vi "globalSetUp.vi"(8 "error in":errorcluster, 11 "Deployment in":refnum<class "Deployment.lvclass">) -> (0 "error out":errorcluster, 3 "Deployment out":refnum<class "Deployment.lvclass">)   [LabVIEW 2020, in "Deployment.lvclass"]
uses:
  Deployment.lvclass
  Shared/Device Parameters.ctl
  Shared/Initialization Method.ctl
  Shared/Bus Selection.ctl
  Shared/Coupling Mode.ctl
  Deployment.lvclass/Deployment.ctl
  niveristand-custom-device-testing-tools/VeriStandTestUtilities/VeriStandTestUtilities.lvlib
  Scripting/AIM MIL-STD-1553 Scripting.lvlib
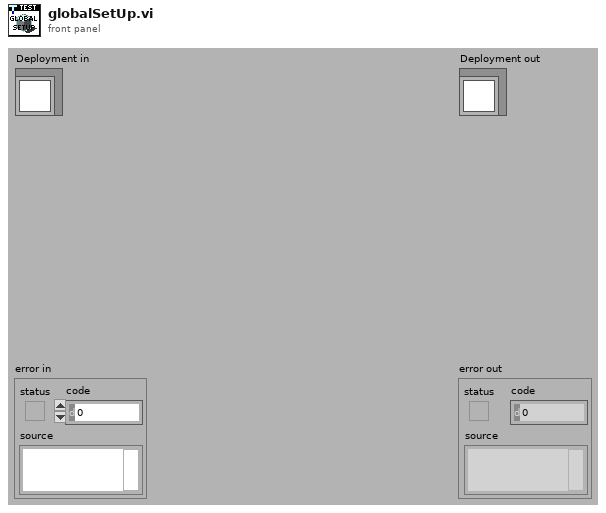
[diagram p1: front panel]
types:
  T1 = typedef "Device Parameters.ctl" = cluster{"initialization method":T2, "card number":i32, "pxi slot number":i32, "biu number":i32, "bus selection":T3, "coupling mode":T4}
  T2 = typedef "Initialization Method.ctl" = enum16{"PXI Slot Number", "Card Number"}
  T3 = typedef "Bus Selection.ctl" = enum16{"Both", "Primary", "Secondary"}
  T4 = typedef "Coupling Mode.ctl" = enum16{"Isolated Onboard Termination", "Transformer Coupled", "Direct Coupled", "External with Onboard Termination", "Onboard Digital Wrap-around"}
  T5 = typedef "Custom Device API.lvlib/Custom Device Item Ref.ctl" = u64
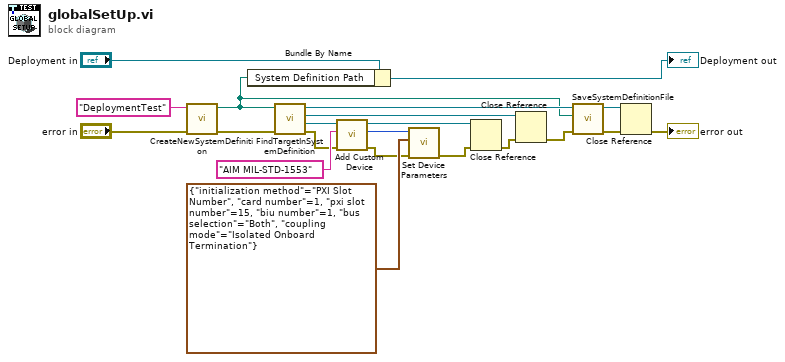
[diagram p0: block diagram]
diagram:
  n1 = call "CreateNewSystemDefinition.vi"("error in"="error in", "System Definition Name"="DeploymentTest") -> ("error out"=w5:errorcluster, "System Definition Path"=w7:path)  [unwired: 8 in]
  n2 = Bundle By Name(cluster="Deployment in", "System Definition Path"=w7) -> (→"Deployment out":refnum<class "Deployment.lvclass">)
  n3 = call "FindTargetInSystemDefinition.vi"("error in"=w5, "system definition path"=w7) -> ("error out"=w12:errorcluster, "Target"=w18:refnum<k24>, "Root"=w17:refnum<k24>, "System Definition"=w19:refnum<k24>)  [unwired: 6 in]
  n4 = call "Add Custom Device.vi"("error in"=w12, "custom device name"="AIM MIL-STD-1553" ("name"), "target"=w18) -> ("error out"=w3:errorcluster, "custom device ref out"=w1:T5, "target out"=w15:refnum<k24>)  [unwired: 6 in]
  n5 = call "Set Device Parameters.vi"("error in"=w3, "device parameters"=T1 {"initialization method"=enum."PXI Slot Number", "card number"=1, "pxi slot number"=15, "biu number"=1, "bus selection"=enum."Both", "coupling mode"=enum."Isolated Onboard Termination"}, "custom device"=w1) -> ("error out"=w2:errorcluster)  [unwired: 7 in, 1 out]
  n6 = Close Reference(reference=w15, error in (no error)=w2) -> (error out=w14:errorcluster)
  n7 = Close Reference(reference=w17, error in (no error)=w14) -> (error out=w16:errorcluster)
  n8 = call "SaveSystemDefinitionFile.vi"("error in (no error)"=w16, "System Definition File in"=w7, "System Definition Reference in"=w19) -> ("error out"=w11:errorcluster, "System Definition Reference out"=w9:refnum<k24>)  [unwired: 7 in]
  n9 = Close Reference(reference=w9, error in (no error)=w11) -> (error out=→"error out":errorcluster)
